vi "Get Outcome.vi"(11 "Test Run Result":refnum<class "Test Run Result.lvclass">) -> (3 "Outcome":T1)   [LabVIEW 2026, in "Test Run Result.lvclass"]
uses:
  Test Run Result.lvclass
  Test Run Result.lvclass/Test Run Result.ctl
  Typedefs/enums/Run Outcome Enum.ctl
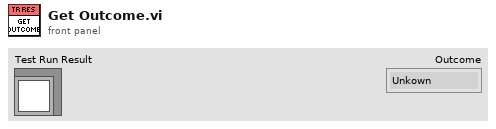
[diagram p1: front panel]
types:
  T1 = typedef "Run Outcome Enum.ctl" = enum16{"Unkown", "Passed", "Failed", "Error", "Aborted"}
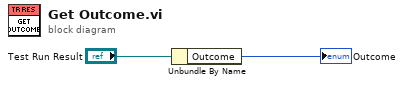
[diagram p0: block diagram]
diagram:
  n1 = Unbundle By Name("Test Run Result") -> ("Outcome"=→"Outcome":T1)
